vi "Scott -- strain -- voltage-wave-form.vi"(10 "time (sec)":dbl, 11 "voltage-parameters-IN":T1) -> (1 "voltage":dbl, 2 "time (sec) out":dbl)   [LabVIEW 2014]
uses:
  FSU/ScottRiggs/Piezo2/voltage-wave-generator-parameters.ctl
panel:
  out "rising lowering":dbl
  out "rising/lowering time":dbl
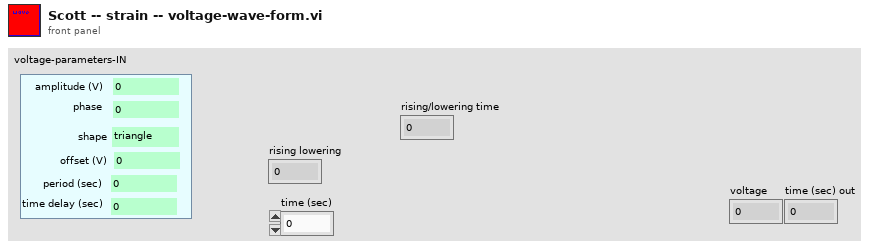
[diagram p1: front panel]
types:
  T1 = typedef "voltage-wave-generator-parameters.ctl" = cluster{"phase ":dbl, "amplitude (V)":dbl, "offset (V)":dbl, "time delay (sec)":dbl, "period (sec)":dbl, "shape":enum16{"triangle", "sine", "none"}}
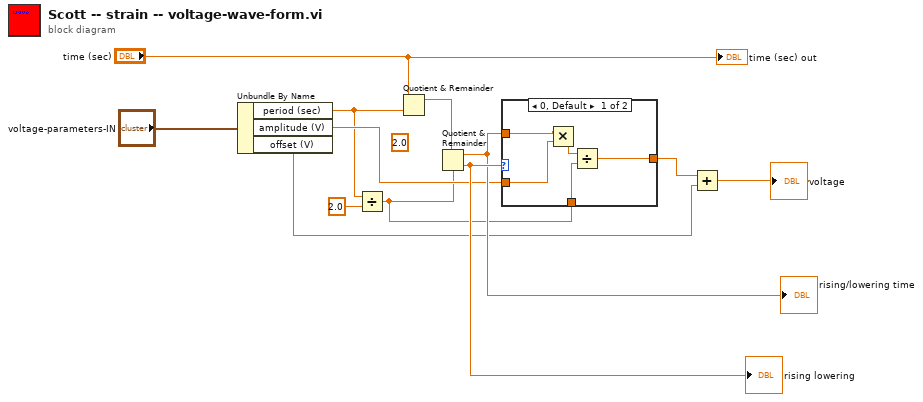
[diagram p0: block diagram]
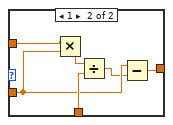
[diagram p2: hidden frame]
diagram:
  (unwired) 2.0 ("y")
  n1 = Unbundle By Name("voltage-parameters-IN") -> ("period (sec)"=w8:dbl, "amplitude (V)"=w9:dbl, "offset (V)"=w5:dbl)
  n2 = Divide(x=w8, y=2.0) -> (x/y=w1:dbl)
  n3 = Quotient & Remainder(x="time (sec)", y=w8) -> (x-y*floor(x/y)=w12:dbl)  [unwired: 1 out]
  n4 = Quotient & Remainder(x=w12, y=w1) -> (x-y*floor(x/y)=w10:dbl, floor(x/y)=w11:dbl)
  "rising/lowering time" <- w10
  "rising lowering" <- w11
  n5 = case shown="0, Default" w11 {
    tunnel: w10 -> [w17 w23]
    tunnel: w9 -> [w16 w20]
    tunnel: w1 -> [w14 w21]
    tunnel: [w13 w18] -> w6
    frame 0, Default {
      n6 = Multiply(x=w17, y=w16) -> (x*y=w15:dbl)
      n7 = Divide(x=w15, y=w14) -> (x/y=w13:dbl)
    }
    frame 1 {
      n8 = Multiply(x=w23, y=w20) -> (x*y=w22:dbl)
      n9 = Divide(x=w22, y=w21) -> (x/y=w19:dbl)
      n10 = Subtract(x=w20, y=w19) -> (x-y=w18:dbl)
    }
  }
  n11 = Add(x=w6, y=w5) -> (x+y=→"voltage":dbl)
  "time (sec) out" <- "time (sec)"
